vi "Get Paths.vi"(7 "Test in":refnum<class "Test.lvclass">, 11 "Path":path) -> (2 "Assert VI Path":path, 3 "Asserts Folder Path":path)   [LabVIEW 2018]
uses:
  Test Classes/Test.lvclass
  Test Classes/Test Class String IDs.vi
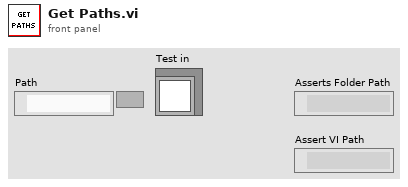
[diagram p1: front panel]
types:
  T1 = cluster{"Comparison Value 1":string, "Comparison Value 2":string, "Invert Result":string, "Assert VI Name":string, "Data Type":string, "Builder User Name":string, "Build Timestamp":string, "Failure Action":string, "Comment":string, "Assert Name":string, "Description":string, "Evaluation String":string}
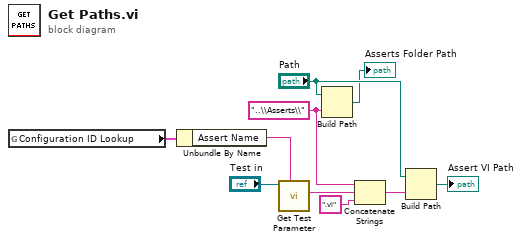
[diagram p0: block diagram]
diagram:
  w6 = "..\\Asserts\\" ("format string")
  n1 = global read "Test Class String IDs.vi" "Configuration ID Lookup"() -> (w4:T1)
  n2 = Unbundle By Name(w4) -> ("Assert Name"=w3:string)
  n3 = call "Get Test Parameter.vi"("Data Value ID"=w3, "Test in"="Test in") -> ("Test Parameter"=w1:string)  [unwired: 7 in, 2 out]
  n4 = Build Path(base path="Path", name or relative path=w6) -> (appended path=→"Asserts Folder Path":path)
  n5 = Concatenate Strings(w6, w1, ".vi" ("format string")) -> (w9:string)
  n6 = Build Path(base path="Path", name or relative path=w9) -> (appended path=→"Assert VI Path":path)
